vi "ReSpaceCode.vi"(11 "Code":string="Script---'''\nhttp://wiki.seeedstudio.com/Grove-LED_Bar/\nhttps://github.com/Seeed-Studio/Grove_LED_Bar/blob/master/Grove_LED_Bar.cpp\nhttps://github.com/Seeed-Studio/Grove_LED_Bar/blob/master/examples/BasicControl/BasicControl.ino\n\nconnections: \nGround (B) - GND \nPower  (R)   - 3V3 \nDCLK (W) - pin Y9\nDIn (Y) -  pin Y10\n'''\n\nimport  utime\nfrom machine import Pin\n\nGLB_CMDMODE = 0x00  # Work on 8-bit mode\n\nclass GroveLEDBar(object):\n    def __init__(self, dio,clk):\n         self.dio = Pin(dio, Pin.OUT,Pin.PULL_UP)\n         self.clk = Pin(clk, Pin.OUT,Pin.PULL_UP)\n\n     def sendData(self,data):\n          state = 0\n          for i in range(16):\n               state1 = (data & 0x8000)\n               self.dio.value(state1)\n               state=1-state\n               self.clk.value(state)\n               data<<=1\n          \n     def latchData(self):\n          self.dio.value(0)\n          utime.sleep_ms(10)\n          for i in range(4):\n               self.dio.value(1)\n               utime.sleep_us(1)\n               self.dio.value(0)\n               utime.sleep_us(1)\n          \n     def setData(self,state):\n          self.sendData(GLB_CMDMODE)\n          for i in range(10):\n               self.sendData(state[i])\n          \n# Two extra empty bits for padding the command to the correct length\n          self.sendData(0x00)\n          self.sendData(0x00)\n          self.latchData(self)\n          \n     def setBits(self,bits):\n          state = bytearray(10)\n          for  i in range(10):\n               if ((bits % 2) == 1):\n                     state[i] = 0xFF\n                else:\n                     state[i] = 0x00\n                bits = int(bits / 2)\n          self.setData(state)\n        \n\nligthts = GroveLEDBar('Y9','Y10')\nlights.setBits(0x3ff)\n") -> (3 "String":string="Script---'''\nhttp://wiki.seeedstudio.com/Grove-LED_Bar/\nhttps://github.com/Seeed-Studio/Grove_LED_Bar/blob/master/Grove_LED_Bar.cpp\nhttps://github.com/Seeed-Studio/Grove_LED_Bar/blob/master/examples/BasicControl/BasicControl.ino\n\nconnections: \nGround (B) - GND \nPower  (R)   - 3V3 \nDCLK (W) - pin Y9\nDIn (Y) -  pin Y10\n'''\n\nimport  utime\nfrom machine import Pin\n\nGLB_CMDMODE = 0x00  # Work on 8-bit mode\n\nclass GroveLEDBar(object):\n     def __init__(self, dio,clk):\n          self.dio = Pin(dio, Pin.OUT,Pin.PULL_UP)\n          self.clk = Pin(clk, Pin.OUT,Pin.PULL_UP)\n\n     def sendData(self,data):\n          state = 0\n          for i in range(16):\n               state1 = (data & 0x8000)\n               self.dio.value(state1)\n               state=1-state\n               self.clk.value(state)\n               data<<=1\n          \n     def latchData(self):\n          self.dio.value(0)\n          utime.sleep_ms(10)\n          for i in range(4):\n               self.dio.value(1)\n               utime.sleep_us(1)\n               self.dio.value(0)\n               utime.sleep_us(1)\n          \n     def setData(self,state):\n          self.sendData(GLB_CMDMODE)\n          for i in range(10):\n               self.sendData(state[i])\n          \n# Two extra empty bits for padding the command to the correct length\n          self.sendData(0x00)\n          self.sendData(0x00)\n          self.latchData(self)\n          \n     def setBits(self,bits):\n          state = bytearray(10)\n          for  i in range(10):\n               if ((bits % 2) == 1):\n                    state[i] = 0xFF\n               else:\n                    state[i] = 0x00\n               bits = int(bits / 2)\n          self.setData(state)\n          \n\nligthts = GroveLEDBar('Y9','Y10')\nlights.setBits(0x3ff)\n")   [LabVIEW 2016]
panel:
  out "Array 2":i32[](array[numeric])
  out "Array":dbl[](array[numeric])=[0.0, 0.0, 0.0, 0.0, 0.0, 0.0, 0.0, 0.0, 0.0, 0.0, 0.0, 0.0, 0.0, 0.0, 0.0, 0.0, 0.0, 0.0, 1.0, 2.0, 2.0, 0.0, 1.0, 2.0, 2.0, 3.0, 3.0, 3.0, 3.0, 3.0, 2.0, 1.0, 2.0, 2.0, 2.0, 3.0, 3.0, 3.0, 3.0, 2.0, 1.0, 2.0, 2.0, 3.0, 2.0, 0.0, 2.0, 2.0, 2.0, 2.0, 1.0, 2.0, 2.0, 3.0, 4.0, 3.0, 4.0, 3.0, 2.0, 2.0, 0.0, 0.0, 0.0]
  out "min value":i32=4
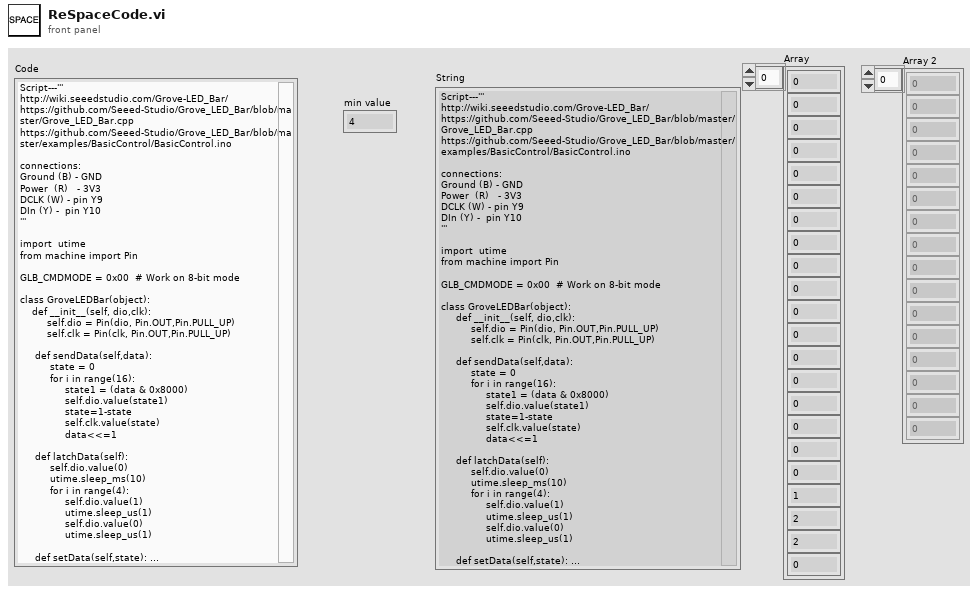
[diagram p1: front panel]
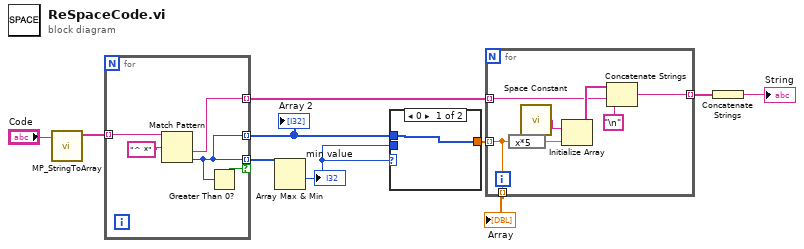
[diagram p0: block diagram]
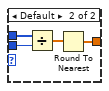
[diagram p2: hidden frame]
diagram:
  n1 = call "MP_StringToArray.vi"("write buffer"="Code") -> ("Array"=w10:string[])  [unwired: 10 in]
  n2 = for {
    tunnel: w10 -> [w14] mode=indexing
    tunnel: [w12] -> w9 mode=indexing if=w13
    tunnel: [w12] -> w8 mode=indexing
    tunnel: [w11] -> w6 mode=indexing
    n3 = Match Pattern(string=w14, regular expression="^ *") -> (after substring=w11:string, offset past match=w12:i32)  [unwired: 1 in, 2 out]
    n4 = Greater Than 0?(x=w12) -> (x > 0?=w13:bool)
  }
  "Array 2" <- w8
  n5 = Array Max & Min(array=w9) -> (min value=w1:i32)  [unwired: 3 out]
  "min value" <- w1
  n6 = case shown="0" w1 {
    tunnel: w8 -> [w16 w20]
    tunnel: [w16 w19] -> w7
    tunnel: w1 -> [_ w17]
    frame 0 {
    }
    frame Default {
      n7 = Divide(x=w20, y=w17) -> (x/y=w18:dbl[])
      n8 = Round To Nearest(number=w18) -> (nearest integer value=w19:dbl[])
    }
  }
  n9 = for {
    tunnel: w7 -> [w21] mode=indexing
    tunnel: w6 -> [w25] mode=indexing
    tunnel: [w22] -> w5 mode=indexing
    tunnel: [w21] -> w2 mode=indexing
    n10 = expression code="x*5"(w21) -> (w24:dbl)
    n11 = call <vilib>:"Space Constant.vi"() -> ("String"=w27:string)
    n12 = Initialize Array(w27, w24) -> (w26:string[])
    n13 = Concatenate Strings(w26, w25, "\n" ("string")) -> (w22:string)
  }
  "Array" <- w2
  n14 = Concatenate Strings(w5) -> (→"String":string)
